vi "내컴퓨터 VI 정보.vi"() -> ()   [LabVIEW 2014]
panel:
  out "배열":string[](array[string])
  in  "머신 IP":string
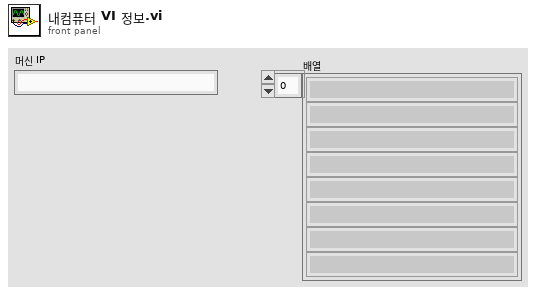
[diagram p1: front panel]
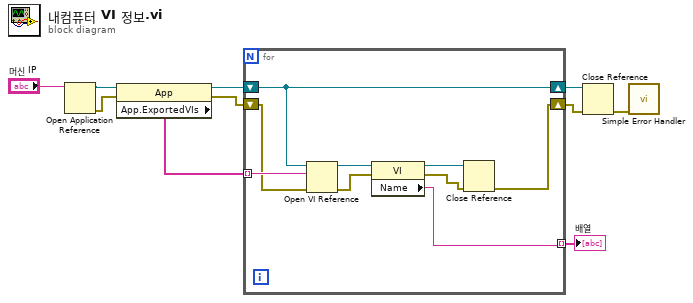
[diagram p0: block diagram]
diagram:
  n1 = Open Application Reference(11:"머신 IP") -> (0:w8:errorcluster, 3:w9:refnum<vi>)  [unwired: 3 in]
  n2 = property class="App"(reference=w9, error in=w8) -> (reference out=w7:refnum<vi>, error out=w6:errorcluster, "App.ExportedVIs"=w5:string[])
  n3 = for {
    shift-right: [w19] -> w2
    shift-left: w7 -> [w19]
    shift-right: [w12] -> w3
    shift-left: w6 -> [w17]
    tunnel: w5 -> [w18] mode=indexing
    tunnel: [w11] -> w4 mode=indexing
    n4 = Open VI Reference(application reference (local)=w19, vi path=w18, error in (no error)=w17) -> (vi reference=w16:refnum<vi>, error out=w15:errorcluster)  [unwired: 3 in]
    n5 = property class="VI"(reference=w16, error in=w15) -> (reference out=w14:refnum<vi>, error out=w13:errorcluster, "Name"=w11:string)
    n6 = Close Reference(reference=w14, error in (no error)=w13) -> (error out=w12:errorcluster)
  }
  "배열" <- w4
  n7 = Close Reference(reference=w2, error in (no error)=w3) -> (error out=w1:errorcluster)
  n8 = call <vilib>:"Simple Error Handler.vi"("error in (no error)"=w1) -> ()  [unwired: 4 in, 5 out]
